vi "Arduino_Upload.vi"(8 "error in (no error)":errorcluster, 10 "VISA resource name":refnum<visa-resource-name>, 11 "Arduino In":T1={"Java"=path "/Applications/Arduino.app/Contents/Java", "Packages"=path "/Users/crogers/Library/Arduino15/packages", "folder"=path "/Users/crogers/Documents/LabVIEW Data", "serial"="/dev/cu.usbmodem14301", "Console"=""}) -> (0 "error out":errorcluster, 3 "Arduino Out":T1={"Java"=path "/Applications/Arduino.app/Contents/Java", "Packages"=path "/Users/crogers/Library/Arduino15/packages", "folder"=path "/Users/crogers/Documents/LabVIEW Data", "serial"="/dev/cu.usbmodem14301", "Console"=""})   [LabVIEW 2020]
uses:
  Arduino.ctl
panel:
  out "resulting string":string
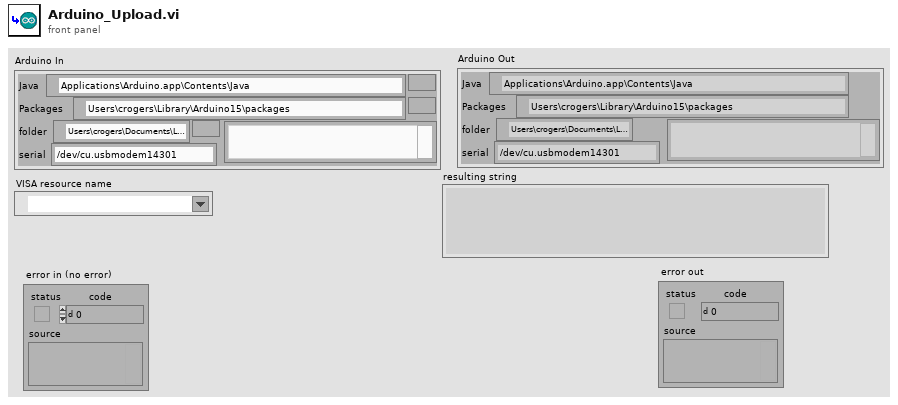
[diagram p1: front panel]
types:
  T1 = typedef "Arduino.ctl" = cluster{"Java":path, "Packages":path, "folder":path, "serial":string, "Console":string}
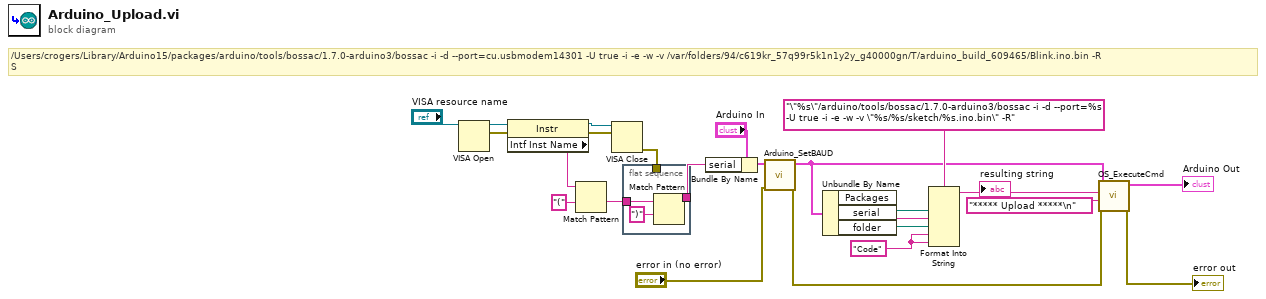
[diagram p0: block diagram]
diagram:
  w11 = "Code" ("Name")
  # "/Users/crogers/Library/Arduino15/packages/arduino/tools/bossac/1.7.0-arduino3/bossac -i -d --port=cu.usbmodem14301 -U true -i -e -w -v /var/folders/94/c619kr_57q99r5k1n1y2y_g40000gn/T/arduino_build_609465/Blink.ino.bin -R \nS"
  n1 = VISA Open(VISA resource name="VISA resource name") -> (VISA resource name=w10:refnum<visa-resource-name>, error out=w3:errorcluster)  [unwired: 4 in]
  n2 = property class="Instr"(reference=w10, error in=w3) -> (reference out=w4:refnum<visa-resource-name>, error out=w2:errorcluster, "Intf Inst Name"=w8:string)
  n3 = Match Pattern(string=w8, regular expression="(") -> (after substring=w6:string)  [unwired: 1 in, 3 out]
  n4 = VISA Close(VISA resource name=w4, error in (no error)=w2) -> (error out=w1:errorcluster)
  n5 = flat-sequence {
    tunnel: w6 -> [w26]
    tunnel: [w25] -> w5
    tunnel: w1 -> [_]
    frame #0 {
      n6 = Match Pattern(string=w26, regular expression=")") -> (before substring=w25:string)  [unwired: 1 in, 3 out]
    }
  }
  n7 = Bundle By Name(cluster="Arduino In", "serial"=w5) -> (w12:T1)
  n8 = call "Arduino_SetBAUD.vi"("error in (no error)"="error in (no error)", "Arduino In"=w12) -> ("error out"=w22:errorcluster, "Arduino Out"=w15:T1)  [unwired: 8 in]
  n9 = Unbundle By Name(w15) -> ("Packages"=w18:path, "serial"=w17:string, "folder"=w16:path)
  n10 = Format Into String(format string="\"%s\"/arduino/tools/bossac/1.7.0-arduino3/bossac -i -d --port=%s -U true -i -e -w -v \"%s/%s/sketch/%s.ino.bin\" -R" ("name or relative path"), w18, w17, w16, w11, w11) -> (resulting string=w20:string)  [unwired: 2 in, 1 out]
  "resulting string" <- w20
  n11 = call "OS_ExecuteCmd.vi"("error in (no error)"=w22, "Comment"="***** Upload *****\n" ("string"), "Command"=w20, "Arduino In"=w15) -> ("error out"=→"error out":errorcluster, "Arduino out"=→"Arduino Out":T1)  [unwired: 6 in]
